vi "CreateTriggerArmNode.vi"(7 "DOM Document":refnum<k20>, 8 "Error In":errorcluster, 11 "Trigger Arm Configuration":T1={"Source"=enum."Hold", "Count"=1, "Infinite?"=FALSE} {"Count" min=1 max=99999 step=1}) -> (0 "Error Out":errorcluster, 3 "Trigger Arm Node":refnum<k20>)   [LabVIEW 2012]
uses:
  TriggerArmConfiguration.ctl
  driver/Public/Controls/ArmSource.ctl
  libs/LV-Utilities/LV-Utilities.lvlib
  driver/Keithley-7001.lvlib
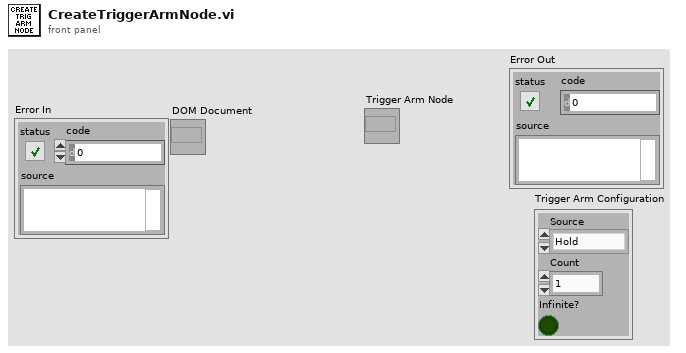
[diagram p1: front panel]
types:
  T1 = typedef "TriggerArmConfiguration.ctl" = cluster{"Source":T2, "Count":u32, "Infinite?":bool}
  T2 = typedef "Keithley-7001.lvlib/ArmSource.ctl" = enum16{"Hold", "Immediate", "Manual", "Bus", "TLink", "External"}
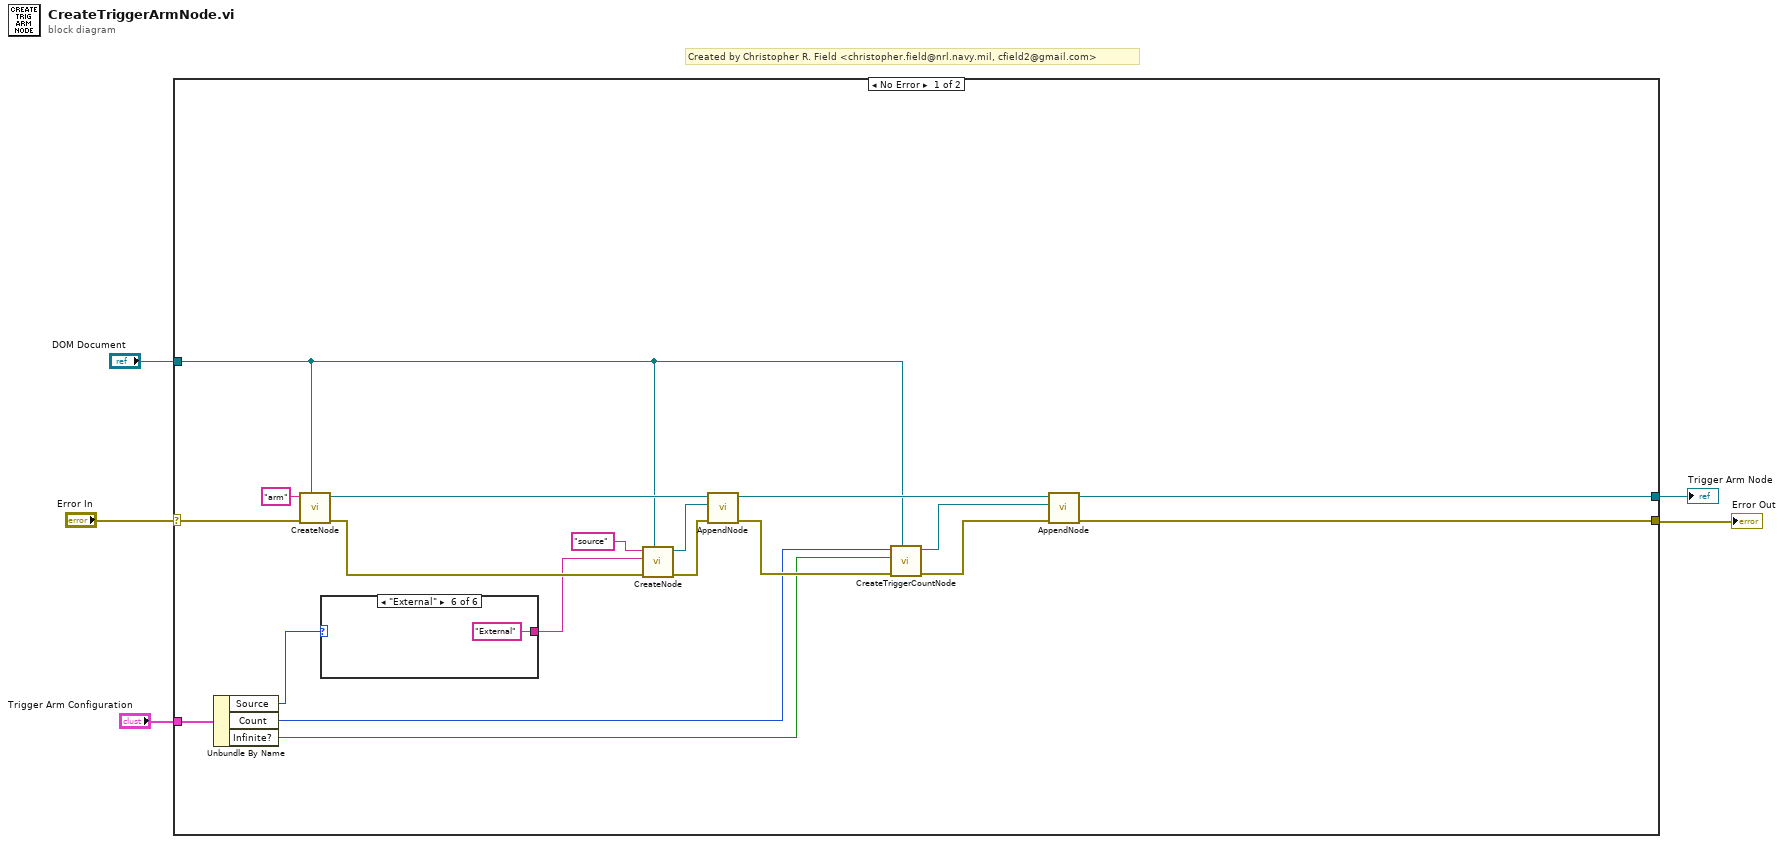
[diagram p0: block diagram]
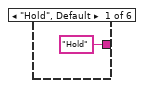
[diagram p2: hidden frame]
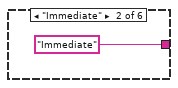
[diagram p3: hidden frame]
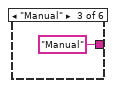
[diagram p4: hidden frame]
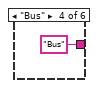
[diagram p5: hidden frame]
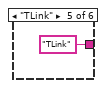
[diagram p6: hidden frame]
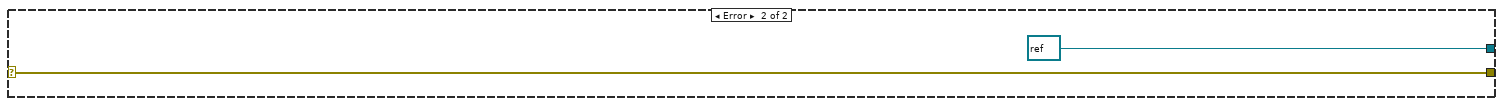
[diagram p7: hidden frame]
diagram:
  # "Created by Christopher R. Field <christopher.field@nrl.navy.mil, cfield2@gmail.com>"
  n1 = case shown="No Error" "Error In" {
    selector: "Error In" -> [w24 w32]
    tunnel: "DOM Document" -> [w9 _]
    tunnel: [w22 w32] -> w3
    tunnel: [w21 refnum<k20> refnum ("Wirings Node 2")] -> w2
    tunnel: "Trigger Arm Configuration" -> [w15 _]
    frame No Error {
      n2 = Unbundle By Name(w15) -> ("Source"=w14:T2, "Count"=w10:u32, "Infinite?"=w8:bool)
      n3 = call "CreateNode.vi"("DOM Document"=w9, "Error In"=w24, "Tag Name"="arm") -> ("Error out"=w19:errorcluster, "Node"=w18:refnum<k20>)  [unwired: 7 in]
      n4 = case shown="\"External\"" w14 {
        tunnel: ["Hold" "Immediate" "Manual" "Bus" "TLink" "External"] -> w13
        frame "Hold", Default {
        }
        frame "Immediate" {
        }
        frame "Manual" {
        }
        frame "Bus" {
        }
        frame "TLink" {
        }
        frame "External" {
        }
      }
      n5 = call "CreateNode.vi"("DOM Document"=w9, "Error In"=w19, "Text"=w13, "Tag Name"="source") -> ("Error out"=w17:errorcluster, "Node"=w16:refnum<k20>)  [unwired: 6 in]
      n6 = call "AppendNode.vi"("Error In"=w17, "Child Node"=w16, "Parent Node In"=w18) -> ("Error Out"=w11:errorcluster, "Parent Node Out"=w12:refnum<k20>)  [unwired: 7 in]
      n7 = call "CreateTriggerCountNode.vi"("DOM Document"=w9, "Error In"=w11, "Infinite?"=w8, "Count"=w10) -> ("Error Out"=w6:errorcluster, "Trigger Count Node"=w7:refnum<k20>)  [unwired: 6 in]
      n8 = call "AppendNode.vi"("Error In"=w6, "Child Node"=w7, "Parent Node In"=w12) -> ("Error Out"=w22:errorcluster, "Parent Node Out"=w21:refnum<k20>)  [unwired: 7 in]
    }
    frame Error {
    }
  }
  "Trigger Arm Node" <- w2
  "Error Out" <- w3
